vi "DL-Flush IPC.vi"(7 "IPC":T1) -> (15 "error out":errorcluster)   [LabVIEW 2020]
uses:
  Typedefs/DL-IPC.ctl
  Typedefs/DL-Configuration.ctl
  Typedefs/DL-Channel Spec.ctl
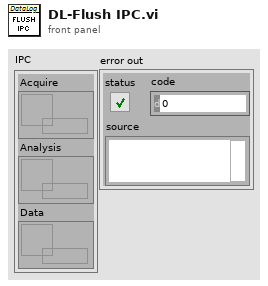
[diagram p1: front panel]
types:
  T1 = typedef "DL-IPC.ctl" = cluster{"Acquire":refnum<queue>, "Analysis":refnum<queue>, "Data":refnum<queue>}
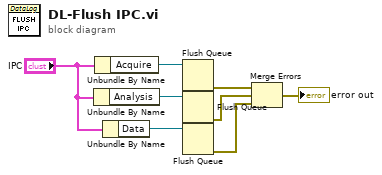
[diagram p0: block diagram]
diagram:
  n1 = Unbundle By Name("IPC") -> ("Analysis"=w5:refnum<queue>)
  n2 = Unbundle By Name("IPC") -> ("Acquire"=w8:refnum<queue>)
  n3 = Unbundle By Name("IPC") -> ("Data"=w4:refnum<queue>)
  n4 = Flush Queue(queue=w8) -> (error out=w7:errorcluster)  [unwired: 1 in, 2 out]
  n5 = Flush Queue(queue=w5) -> (error out=w2:errorcluster)  [unwired: 1 in, 2 out]
  n6 = Flush Queue(queue=w4) -> (error out=w1:errorcluster)  [unwired: 1 in, 2 out]
  n7 = Merge Errors(w7, w2, w1) -> (→"error out":errorcluster)
